vi "SRV_Write Sensor Commands.vi"(0 "SRV In":refnum<k5>, 5 "Sensor Cfg-Commands":T1[](array[typedef]) {"Calculated Sensors Array"."Parsed Formula"."Y Values" format="%.2f"; "Calculated Sensors Array"."Sensor Config"."Register" format="%.0x"; "Calculated Sensors Array"."Sensor Config"."I2C Address" format="%.0x"; "Calculated Sensors Array"."Sensor Config"."Sample Period (ms)" min=10 max=60000 step=1; "Calculated Sensors Array"."Sensor Config"."Digital Mask" format="%.0x"; "Calculated Sensors Array"."Sensor Config"."Channel" format="%.0x"; "Parsed Formula"."Y Values" format="%.2f"; "Sensor Config"."Register" format="%.0x"; "Sensor Config"."I2C Address" format="%.0x"; "Sensor Config"."Sample Period (ms)" min=10 max=60000 step=1; "Sensor Config"."Digital Mask" format="%.0x"; "Sensor Config"."Channel" format="%.0x"}, 11 "error in (no error)":errorcluster) -> (4 "SRV out":refnum<k5>, 15 "error out":errorcluster)   [LabVIEW 2014]
uses:
  SRV_Sensor Config-Command Cluster.ctl
  SRV_Sensor Config Cluster.ctl
  SRV_Sensor Analog-Digital.ctl
  SRV_Sensor Sampling Mode.ctl
  SRV_Sensor View Config Cluster.ctl
  SRV_Sensors Names.ctl
  SRV_Sensor PicoC Shared Var Type.ctl
  SRV_Sensor Number of Bytes.ctl
  SRV_Sensor Integer Word Type.ctl
  SRV_Calculated Sensor Cfg.ctl
panel:
  # "operator"
  # "register1"
  # "register2"
  # "operator"
  # "register1"
  # "register2"
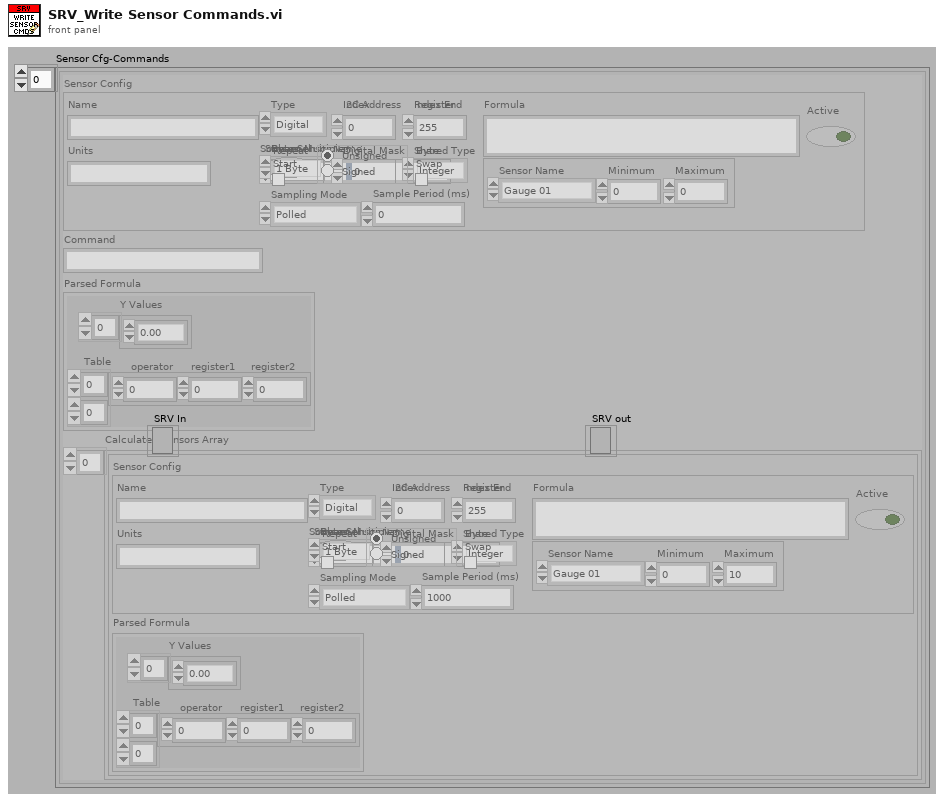
[diagram p1: front panel]
types:
  T1 = typedef "SRV_Sensor Config-Command Cluster.ctl" = cluster{"Sensor Config":T2, "Command":string, "Parsed Formula":cluster{"Table":i32[][], "Y Values":dbl[]}, "Calculated Sensors Array":T10[]}
  T2 = typedef "SRV_Sensor Config Cluster.ctl" = cluster{"Name":string, "A/D":T3, "I2C Address":u8, "Register":u8, "Channel":u8, "Digital Mask":u16, "Units":string, "Sampling Mode":T4, "Sample Period (ms)":u32, "Formula":string, "Sensor View Config":T5, "Active":bool, "PicoC Shared Var Type":T7, "Index":u8, "Stream Multiple?":bool, "Index End":u8, "Bytes":T8, "Source Sensor Name":string, "Repeat Start":bool, "Integer Word Type":T9, "Byte Swap":bool}
  T3 = typedef "SRV_Sensor Analog-Digital.ctl" = enum16{"Digital", "Analog", "PicoC Shared", "Calculated"}
  T4 = typedef "SRV_Sensor Sampling Mode.ctl" = enum16{"Polled", "Streaming"}
  T5 = typedef "SRV_Sensor View Config Cluster.ctl" = cluster{"Sensor Name":T6, "Minimum":dbl, "Maximum":dbl}
  T6 = typedef "SRV_Sensors Names.ctl" = enum16{"Gauge 01", "Gauge 02", "Gauge 03", "Gauge 04", "Meter 01", "Meter 02", "Meter 03", "Meter 04", "Numeric 01", "Numeric 02", "Numeric 03", "Numeric 04", "Numeric 05", "Numeric 06", "Numeric 07", "Numeric 08", "Boolean 01", "Boolean 02", "Boolean 03", "Boolean 04", "Boolean 05", "Boolean 06", "Boolean 07", "Boolean 08", "Boolean 09", "Boolean 10", "Boolean 11", "Boolean 12", "Boolean 13", "Boolean 14", "Boolean 15", "Boolean 16", "Boolean 17", "Boolean 18", "Boolean 19", "Boolean 20", "Boolean 21", "Boolean 22", "Boolean 23", "Boolean 24", "Boolean 25", "Boolean 26", "Boolean 27", "Boolean 28", "Boolean 29", "Boolean 30", "Boolean 31", "Boolean 32"}
  T7 = typedef "SRV_Sensor PicoC Shared Var Type.ctl" = enum16{"String", "Integer", "Float"}
  T8 = typedef "SRV_Sensor Number of Bytes.ctl" = enum16{"1 Byte", "2 Bytes"}
  T9 = typedef "SRV_Sensor Integer Word Type.ctl" = enum32{"Unsigned", "Signed"}
  T10 = typedef "SRV_Calculated Sensor Cfg.ctl" = cluster{"Sensor Config":T2, "Parsed Formula":cluster{"Table":i32[][], "Y Values":dbl[]}}
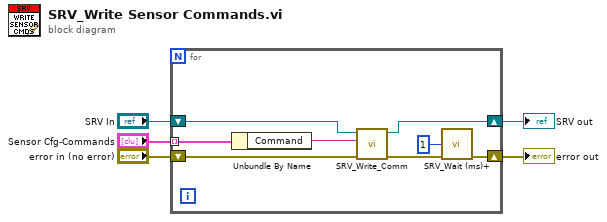
[diagram p0: block diagram]
diagram:
  n1 = for {
    tunnel: "Sensor Cfg-Commands" -> [w12] mode=indexing
    shift-right: [w7] -> w2
    shift-left: "error in (no error)" -> [w10]
    shift-right: [w9] -> w1
    shift-left: "SRV In" -> [w13]
    n2 = Unbundle By Name(w12) -> ("Command"=w11:string)
    n3 = call "SRV_Write_Comm.vi"("error in (no error)"=w10, "Command Sent"=w11, "SRV In"=w13) -> ("error out"=w8:errorcluster, "SRV Out"=w9:refnum<k5>)  [unwired: 6 in, 1 out]
    n4 = call "SRV_Wait (ms)+.vi"("milliseconds to wait"=u32 1, "error in (no error)"=w8) -> ("error out"=w7:errorcluster)  [unwired: 12 in, 1 out]
  }
  "error out" <- w2
  "SRV out" <- w1
